vi "Read Location.vi"(8 "error in (no error)":errorcluster, 11 "FSM.Port in":refnum<class "FSM.Port.lvclass">) -> (0 "error out":errorcluster, 2 "Location":cluster{"x":i16, "y":i16}, 3 "FSM.Port out":refnum<class "FSM.Port.lvclass">)   [LabVIEW 2020, in "FSM.Port.lvclass"]
uses:
  FSM.Port.lvclass
  FSM.Port.lvclass/FSM.Port.ctl
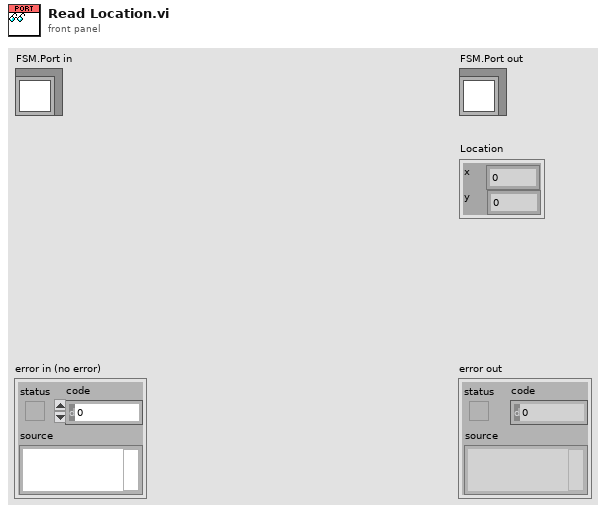
[diagram p1: front panel]
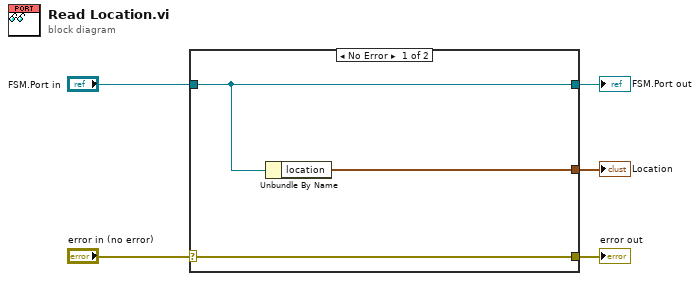
[diagram p0: block diagram]
diagram:
  n1 = case shown="No Error" "error in (no error)" {
    selector: "error in (no error)" -> [w8 w9]
    tunnel: [w8 w9] -> w4
    tunnel: [w7 w10] -> w2
    tunnel: "FSM.Port in" -> [w7 w10]
    tunnel: [w6 _] -> w1
    frame No Error {
      n2 = Unbundle By Name(w7) -> ("location"=w6:cluster{"x":i16, "y":i16})
    }
    frame Error {
    }
  }
  "error out" <- w4
  "FSM.Port out" <- w2
  "Location" <- w1
